vi "ep_Error Checking.vi"(7 "reset? (F)":bool, 8 "error in (no error)":errorcluster, 9 "system info in":refnum<class "EP System Info.lvclass">, 10 "reference channel index":i32, 11 "data":waveform(dbl)[](array[waveform])) -> (0 "error out":errorcluster, 1 "system info out":refnum<class "EP System Info.lvclass">, 2 "t0":timestamp, 3 "signals":dbl[][](array[numeric]), 5 "dt":dbl)   [LabVIEW 2013, in "NI_EP_Resample_Host.lvlib"]
uses:
  <vilib>/addons/Electrical Power/PQ/Resampling/NI_EP_Resample_Host.lvlib
  <vilib>/addons/Electrical Power/PQ/Common/Classes/System Info/EP System Info.lvclass
  <vilib>/addons/Electrical Power/Power Measurement/NI_EP_Power Measurement.lvlib
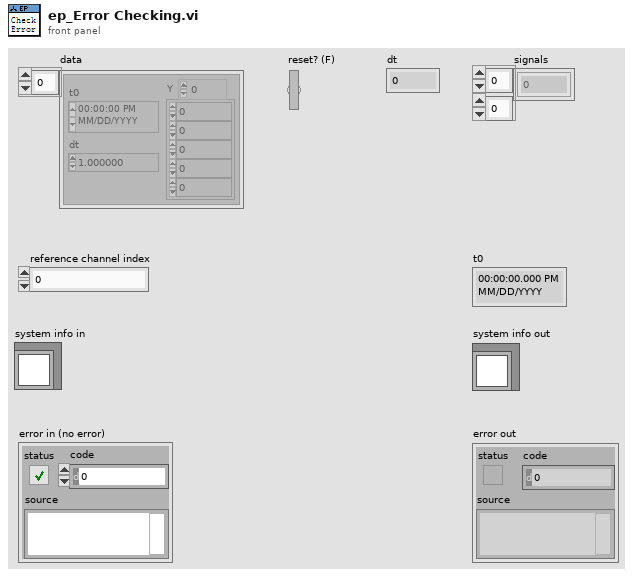
[diagram p1: front panel]
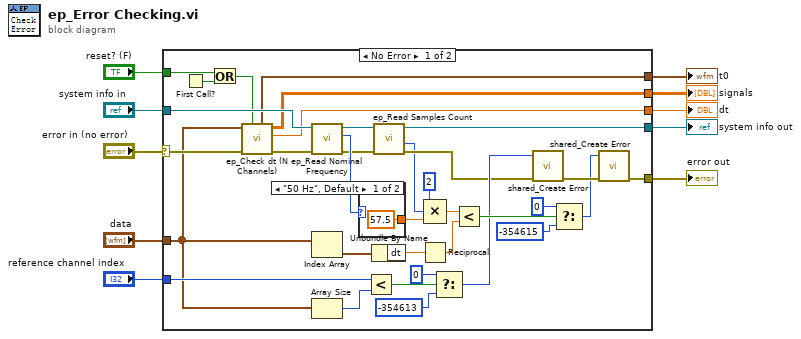
[diagram p0: block diagram]
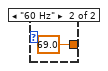
[diagram p2: hidden frame]
diagram:
  n1 = case shown="No Error" "error in (no error)" {
    selector: "error in (no error)" -> [w19 w47]
    tunnel: "reference channel index" -> [w44 _]
    tunnel: [w37 w47] -> w9
    tunnel: "data" -> [w17 _]
    tunnel: "system info in" -> [w30 w48]
    tunnel: [w27 w48] -> w7
    tunnel: [w16 _] -> w4
    tunnel: [w15 _] -> w3
    tunnel: [w14 _] -> w2
    tunnel: "reset? (F)" -> [w11 _]
    frame No Error {
      n2 = First Call?() -> (First Call?: T/F=w12:bool)
      n3 = Or(x=w11, y=w12) -> (x .or. y?=w13:bool)
      n4 = call <vilib>:"ep_Check dt (N Channels).vi"("reset? (F)"=w13, "error in (no error)"=w19, "waveforms"=w17) -> ("error out"=w18:errorcluster, "dt"=w14:dbl, "signals"=w15:dbl[][], "t0"=w16:timestamp)  [unwired: 4 in, 1 out]
      n5 = call <vilib>:"ep_Read Nominal Frequency.vi"("error in (no error)"=w18, "system info in"=w30) -> ("error out"=w24:errorcluster, "nominal frequency"=w29:enum16{"50 Hz", "60 Hz"}, "system info out"=w28:refnum<class "EP System Info.lvclass">)  [unwired: 6 in, 1 out]
      n6 = Index Array(array=w17) -> (element=w39:waveform(dbl))  [unwired: 1 in]
      n7 = Array Size(array=w17) -> (size(s)=w43:i32)
      n8 = case shown="\"50 Hz\", Default" w29 {
        tunnel: [57.5 69.0] -> w20
        frame "50 Hz", Default {
        }
        frame "60 Hz" {
        }
      }
      n9 = Less?(x=w44, y=w43) -> (x < y?=w42:bool)
      n10 = Unbundle By Name(w39) -> ("dt"=w33:dbl)
      n11 = call <vilib>:"ep_Read Samples Count.vi"("error in (no error)"=w24, "system info in"=w28) -> ("error out"=w23:errorcluster, "half-cycle (samples)"=w22:i32, "system info out"=w27:refnum<class "EP System Info.lvclass">)  [unwired: 5 in, 2 out]
      n12 = Reciprocal(x=w33) -> (1/x=w32:dbl)
      n13 = Compound Arithmetic op=MULTIPLY(2 ("value"), w22, w20) -> (w34:dbl)
      n14 = Select(t=0, s=w42, f=-354613) -> (s? t:f=w25:i32)
      n15 = Less?(x=w34, y=w32) -> (x < y?=w31:bool)
      n16 = call <vilib>:"shared_Create Error.vi"("error in (no error)"=w23, "error code (0)"=w25) -> ("error out"=w38:errorcluster)  [unwired: 9 in]
      n17 = Select(t=0, s=w31, f=-354615) -> (s? t:f=w26:i32)
      n18 = call <vilib>:"shared_Create Error.vi"("error in (no error)"=w38, "error code (0)"=w26) -> ("error out"=w37:errorcluster)  [unwired: 9 in]
    }
    frame Error {
    }
  }
  "error out" <- w9
  "system info out" <- w7
  "t0" <- w4
  "signals" <- w3
  "dt" <- w2
